vi "Get Protocol List.vi"(8 "error in (no error)":errorcluster) -> (0 "error out":errorcluster, 3 "Class Lookup":variant)   [LabVIEW 2019, in "Instrument Addon Shared.lvlib"]
uses:
  Instrument Addon Shared.lvlib
  <vilib>/Utility/LVLibp/NI_PackedLibraryUtility.lvlib
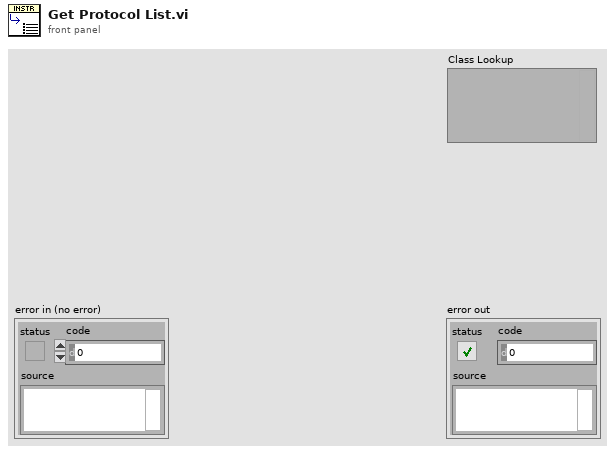
[diagram p1: front panel]
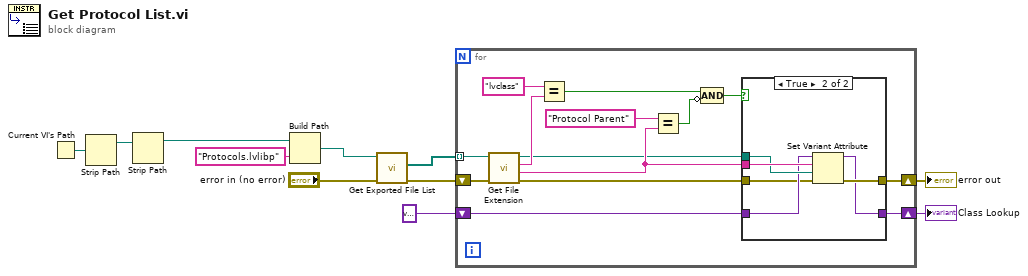
[diagram p0: block diagram]
diagram:
  n1 = Current VI's Path() -> (path=w11:path)
  n2 = Strip Path(path=w11) -> (stripped path=w10:path)  [unwired: 1 out]
  n3 = Strip Path(path=w10) -> (stripped path=w9:path)  [unwired: 1 out]
  n4 = Build Path(base path=w9, name or relative path="Protocols.lvlibp") -> (appended path=w1:path)
  n5 = call <vilib>:"Get Exported File List.vi"("error in (no error)"="error in (no error)", "packed library path"=w1) -> ("error out"=w6:errorcluster, "paths"=w7:path[])  [unwired: 7 in, 1 out]
  n6 = for {
    tunnel: w7 -> [w20] mode=indexing
    shift-right: [w14] -> w4
    shift-left: w6 -> [w21]
    shift-right: [w13] -> w3
    shift-left: variant ("variant") -> [w16]
    n7 = call <vilib>:"Get File Extension.vi"("error in (no error)"=w21, "file"=w20) -> ("error out"=w15:errorcluster, "filename without extension"=w18:string, "lowercase file extension"=w22:string, "dup file"=w17:path)  [unwired: 5 in, 1 out]
    n8 = Equal?(x="lvclass" ("string"), y=w22) -> (x = y?=w24:bool)
    n9 = Equal?(x="Protocol Parent", y=w18) -> (x = y?=w19:bool)
    n10 = Compound Arithmetic op=AND(w24, invert w19) -> (w12:bool)
    n11 = case shown="True" w12 {
      tunnel: w18 -> [_ w33]
      tunnel: w17 -> [_ w32]
      tunnel: w16 -> [w26 w31]
      tunnel: w15 -> [w27 w30]
      tunnel: [w27 w29] -> w14
      tunnel: [w26 w28] -> w13
      frame False {
      }
      frame True {
        n12 = Set Variant Attribute(Variant=w31, name=w33, value=w32, error in=w30) -> (Variant out=w28:variant, error out=w29:errorcluster)  [unwired: 1 out]
      }
    }
  }
  "error out" <- w4
  "Class Lookup" <- w3
